vi "Assisted Turning.vi"(2 "Left":bool, 3 "Current Value":dbl format="%#_13g", 4 "Right":bool, 5 "Turn Amount":dbl=90.0 format="%#_13g") -> (0 "New Value":dbl format="%#_13g", 1 "Same Target":bool)   [LabVIEW 2016, in "ArgosLib.lvlib"]
uses:
  ArgosLib.lvlib
  Signal Processing/TypeDefs/EdgeDetector_Type.ctl
panel:
  # "Increments or decrements a value by a given amount on buton presses.\nUseful to step through rotational positions clockwise/counterclockwise"
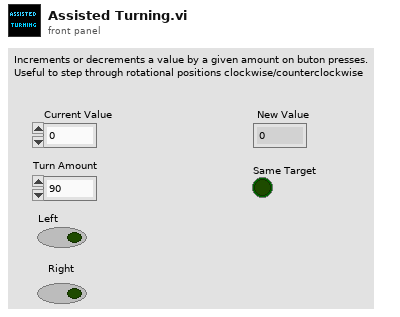
[diagram p1: front panel]
types:
  T1 = typedef "EdgeDetector_Type.ctl" = enum16{"RisingEdge", "FallingEdge", "Both"}
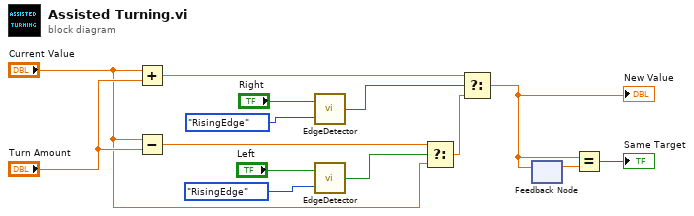
[diagram p0: block diagram]
diagram:
  n1 = Add(x="Current Value", y="Turn Amount") -> (x+y=w11:dbl)
  n2 = Subtract(x="Current Value", y="Turn Amount") -> (x-y=w12:dbl)
  n3 = call "EdgeDetector.vi"("DetectorType"=EdgeDetector_Type."RisingEdge", "Input"="Right") -> ("Edge"=w1:bool)
  n4 = call "EdgeDetector.vi"("DetectorType"=EdgeDetector_Type."RisingEdge", "Input"="Left") -> ("Edge"=w6:bool)
  n5 = Select(t=w12, s=w6, f="Current Value") -> (s? t:f=w14:dbl)
  n6 = Select(t=w11, s=w1, f=w14) -> (s? t:f=w7:dbl)
  "New Value" <- w7
  n7 = feedback-in #1(w7) -> ()
  n8 = feedback #1() -> (w8:dbl)  [unwired: 1 in]
  n9 = Equal?(x=w7, y=w8) -> (x = y?=→"Same Target":bool)
